vi "RemoveValue.vi"(5 "Input aArray":dbl[](array[numeric]), 9 "Valeur à enlever":dbl=255.0) -> (6 "Output Array":dbl[](array[numeric]))   [LabVIEW 2019]
panel:
  out "Nb_rm":i32
  out "ExecTime":u32
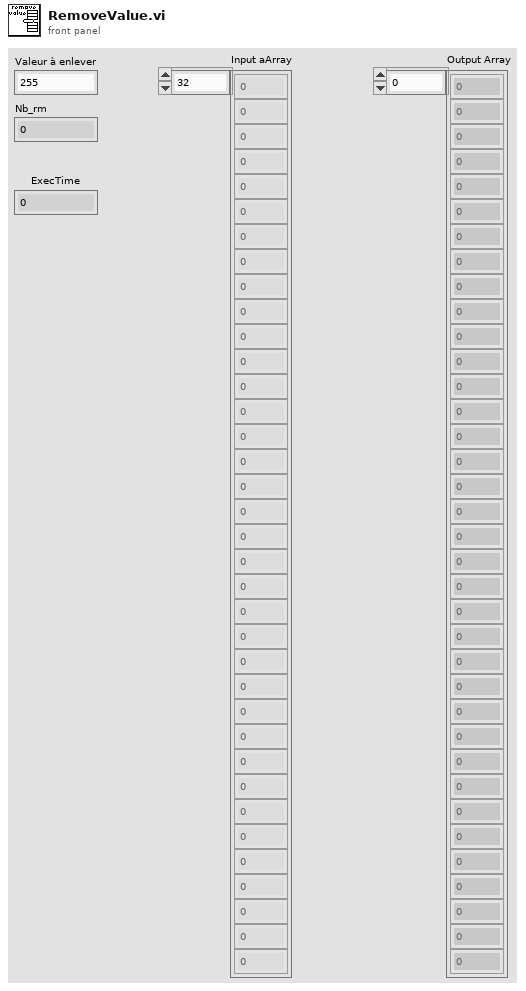
[diagram p1: front panel]
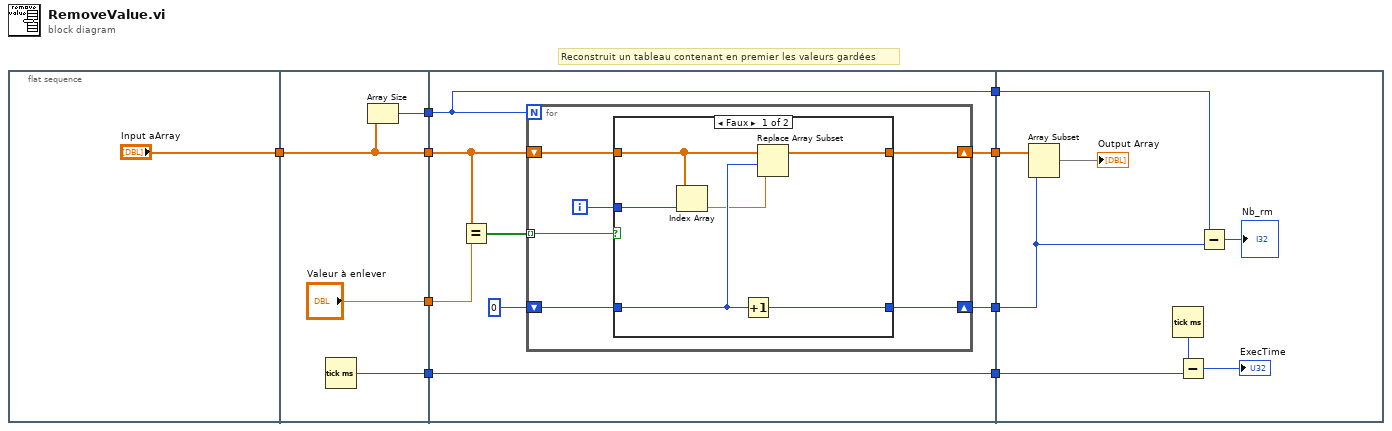
[diagram p0: block diagram]
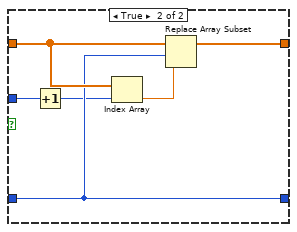
[diagram p2: hidden frame]
diagram:
  # "Reconstruit un tableau contenant en premier les valeurs gardées"
  n1 = flat-sequence {
    tunnel: ["Input aArray"] -> w9
    tunnel: w9 -> [w12]
    tunnel: [w12] -> w8
    tunnel: ["Valeur à enlever"] -> w7
    tunnel: [w13] -> w5
    tunnel: [w11] -> w2
    tunnel: w8 -> [w20]
    tunnel: w7 -> [w22]
    tunnel: [w21] -> w6
    tunnel: w5 -> [w21]
    tunnel: [w17] -> w4
    tunnel: [w16] -> w3
    tunnel: w2 -> [w15]
    tunnel: [w15] -> w1
    tunnel: w6 -> [w48]
    tunnel: w4 -> [w45]
    tunnel: w3 -> [w43]
    tunnel: w1 -> [w42]
    frame #0 {
    }
    frame #1 {
      n2 = Tick Count (ms)() -> (millisecond timer value=w13:u32)
      n3 = Array Size(array=w12) -> (size(s)=w11:i32)
    }
    frame #2 {
      n4 = Equal?(x=w20, y=w22) -> (x = y?=w19:bool[])
      n5 = for {
        N: w15 -> [_]
        tunnel: w19 -> [w28] mode=indexing
        shift-right: [w24] -> w17
        shift-left: w20 -> [w27]
        shift-right: [w25] -> w16
        shift-left: 0 ("Nb Zeros") -> [w26]
        i -> [w23]
        n6 = case shown="Faux" w28 {
          tunnel: w27 -> [w29 w38]
          tunnel: w26 -> [w31 w36]
          tunnel: [w34 w36] -> w25
          tunnel: [w33 w40] -> w24
          tunnel: w23 -> [w32 w37]
          frame False {
            n7 = Index Array(array=w29, index=w32) -> (element=w30:dbl)
            n8 = Increment(x=w31) -> (x+1=w34:i32)
            n9 = Replace Array Subset(array=w29, new element=w30, index=w31) -> (w33:dbl[])
          }
          frame True {
            n10 = Increment(x=w37) -> (x+1=w35:i32)
            n11 = Index Array(array=w38, index=w35) -> (element=w39:dbl)
            n12 = Replace Array Subset(array=w38, new element=w39, index=w36) -> (w40:dbl[])
          }
        }
      }
    }
    frame #3 {
      n13 = Array Subset(array=w45, length=w43) -> (→"Output Array":dbl[])  [unwired: 1 in]
      n14 = Tick Count (ms)() -> (millisecond timer value=w47:u32)
      n15 = Subtract(x=w47, y=w48) -> (x-y=→"ExecTime":u32)
      n16 = Subtract(x=w42, y=w43) -> (x-y=→"Nb_rm":i32)
    }
  }
